vi "Set conversion_units.vi"(8 "error in (no error)":errorcluster, 11 "DLOwis in":refnum<class "DLOwis.lvclass">) -> (0 "error out":errorcluster, 1 "Velocities":dbl[](array[numeric]), 2 "pitches":dbl[](array[numeric]), 3 "DLOwis out":refnum<class "DLOwis.lvclass">)   [LabVIEW 2020, in "DLOwis.lvclass"]
uses:
  DLOwis.lvclass
  C:/Dev/TRANCON/Classes/GeneralFunctionality/GeneralFunctionality.lvclass
  GeneralFunctionality/GeneralFunctionality.lvclass/GeneralFunctionality.ctl
  Config/Config.lvclass
  DLOwis.lvclass/DLOwis.ctl
  GeneralFunctionality/GeneralFunctionality.lvclass
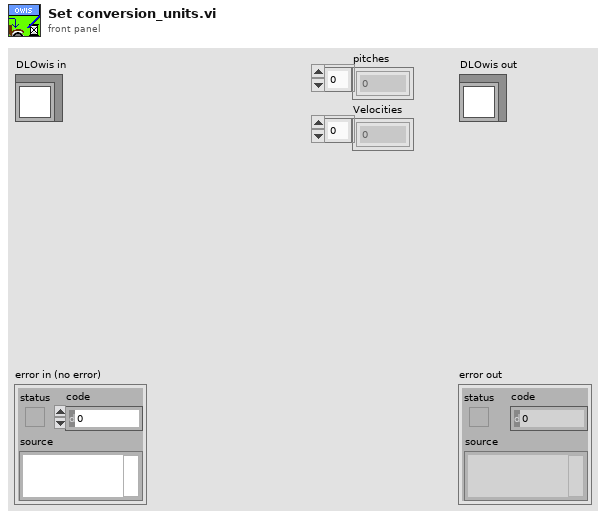
[diagram p1: front panel]
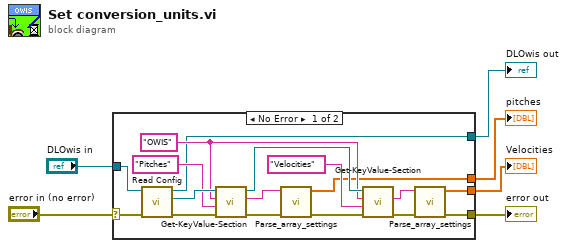
[diagram p0: block diagram]
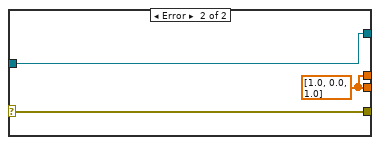
[diagram p2: hidden frame]
diagram:
  n1 = case shown="No Error" "error in (no error)" {
    selector: "error in (no error)" -> [w23 w26]
    tunnel: [w13 w26] -> w3
    tunnel: [w7 w25] -> w4
    tunnel: "DLOwis in" -> [w17 w25]
    tunnel: [w9 w24] -> w2
    tunnel: [w8 w24] -> w1
    frame No Error {
      w11 = "OWIS" ("Section")
      n2 = call "Read Config.vi"("error in (no error)"=w23, "GeneralFunctionality en entrée"=w17) -> ("error out"=w22:errorcluster, "Config.lvclass"=w21:refnum<class "Config.lvclass">, "GeneralFunctionality en sortie"=w7:refnum<class "DLOwis.lvclass">)  [unwired: 7 in]
      n3 = call-dynamic "Get-KeyValue-Section.vi"("error in (no error)"=w22, "Key"="Pitches", "Section"=w11, "Config in"=w21) -> ("error out"=w19:errorcluster, "Value"=w18:string, "Config out"=w16:refnum<class "Config.lvclass">)  [unwired: 5 in]
      n4 = call "Parse_array_settings.vi"("error in (no error)"=w19, "Value"=w18) -> ("error out"=w15:errorcluster, "Array"=w8:dbl[])  [unwired: 8 in]
      n5 = call-dynamic "Get-KeyValue-Section.vi"("error in (no error)"=w15, "Key"="Velocities", "Section"=w11, "Config in"=w16) -> ("error out"=w14:errorcluster, "Value"=w12:string)  [unwired: 5 in, 1 out]
      n6 = call "Parse_array_settings.vi"("error in (no error)"=w14, "Value"=w12) -> ("error out"=w13:errorcluster, "Array"=w9:dbl[])  [unwired: 8 in]
    }
    frame Error {
      w24 = dbl[] [1.0, 0.0, 1.0] ("Array")
    }
  }
  "error out" <- w3
  "DLOwis out" <- w4
  "Velocities" <- w2
  "pitches" <- w1
